vi "Square Clock DUPE subVI.vi"(8 "Last Bool State":bool, 9 "Sample Rate (Hz)":dbl, 10 "SampleDelay(in)":u32=1000, 11 "Last Event mS":u32) -> (0 "Clock Output":bool, 3 "Last Event mS":u32, 4 "Elapsed mS":u32, 6 "SampleDelay":u32)   [LabVIEW 2021]
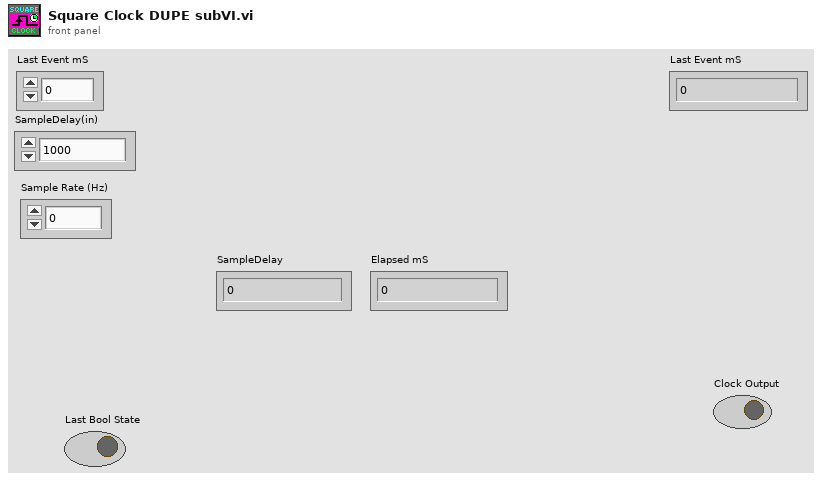
[diagram p1: front panel]
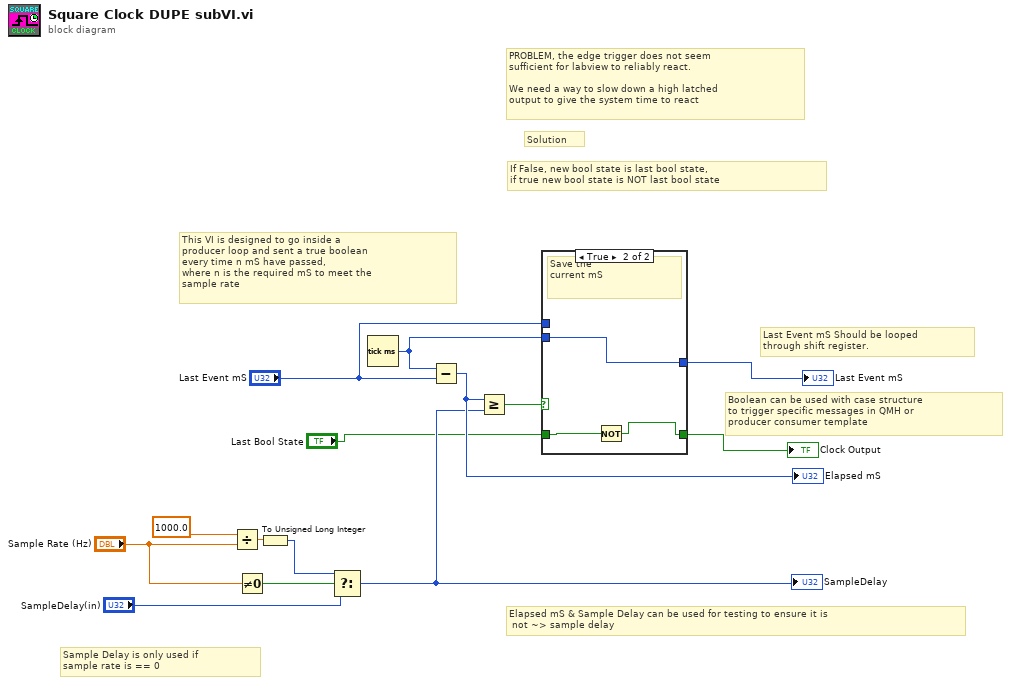
[diagram p0: block diagram]
diagram:
  # "Solution"
  # "If False, new bool state is last bool state,\nif true new bool state is NOT last bool state"
  # "PROBLEM, the edge trigger does not seem \nsufficient for labview to reliably react.\n\nWe need a way to slow down a high latched \noutput to give the system time to react"
  # "Sample Delay is only used if\nsample rate is == 0"
  # "Elapsed mS & Sample Delay can be used for testing to ensure it is\n not ~> sample delay"
  # "Boolean can be used with case structure\nto trigger specific messages in QMH or \nproducer consumer template"
  # "This VI is designed to go inside a\nproducer loop and sent a true boolean\nevery time n mS have passed, \nwhere n is the required mS to meet the \nsample rate"
  # "Last Event mS Should be looped\nthrough shift register."
  n1 = Divide(x=1000.0, y="Sample Rate (Hz)") -> (x/y=w12:dbl)
  n2 = Not Equal To 0?(x="Sample Rate (Hz)") -> (x != 0?=w9:bool)
  n3 = To Unsigned Long Integer(number=w12) -> (unsigned 32bit integer=w8:u32)
  n4 = Select(t=w8, s=w9, f="SampleDelay(in)") -> (s? t:f=w2:u32)
  "SampleDelay" <- w2
  n5 = Tick Count (ms)() -> (millisecond timer value=w3:u32)
  n6 = Subtract(x=w3, y="Last Event mS") -> (x-y=w6:u32)
  "Elapsed mS" <- w6
  n7 = Greater Or Equal?(x=w6, y=w2) -> (x >= y?=w5:bool)
  n8 = case shown="True" w5 {
    tunnel: [w16 w19] -> w13
    tunnel: w3 -> [_ w19]
    tunnel: "Last Event mS" -> [w16 _]
    tunnel: [w15 w17] -> w14
    tunnel: "Last Bool State" -> [w15 w18]
    frame False {
      # "Keep Checking\nAgainst\nLast mS"
    }
    frame True {
      # "Save the \ncurrent mS"
      n9 = Not(x=w18) -> (.not. x?=w17:bool)
    }
  }
  "Last Event mS" <- w13
  "Clock Output" <- w14
